vi "Start Module.vi"   [LabVIEW 2020]
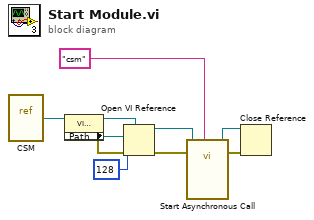
[diagram p0: block diagram]
diagram:
  n1 = vi-ref "CSM.vi"() -> (w4:refnum<vi>)
  n2 = property class="VI (strict)"(reference=w4) -> (reference out=w8:refnum<vi>, error out=w6:errorcluster, "Path"=w5:path)  [unwired: 1 in]
  n3 = Open VI Reference(type specifier VI Refnum (for type only)=w8, vi path=w5, options=128, error in (no error)=w6) -> (vi reference=w3:refnum<vi>, error out=w9:errorcluster)  [unwired: 2 in]
  n4 = call-by-ref "Start Asynchronous Call"(reference=w3, error in=w9, "Name(\"\" to use uuid)"="csm" ("Name(\"\" to use uuid)")) -> (reference out=w2:refnum<vi>, error out=w7:errorcluster)  [unwired: 11 in]
  n5 = Close Reference(reference=w2, error in (no error)=w7) -> ()  [unwired: 1 out]
